vi "GetSpicyPizza.vi"(8 "error in (no error)":errorcluster, 11 "Waiter(Director) in":refnum<class "Waiter(Director).lvclass">) -> (0 "error out":errorcluster, 2 "Pizza":refnum<class "Pizza(Product).lvclass">, 3 "Waiter(Director) out":refnum<class "Waiter(Director).lvclass">)   [LabVIEW 2014, in "Waiter(Director).lvclass"]
uses:
  Waiter(Director).lvclass
  Pizza(Product)/Pizza(Product).lvclass
  ConcreteBuilder/SpicyPizzaBuilder/SpicyPizzaBuilder.lvclass
  Cook(builder)/PizzaBuilder(Builder).lvclass
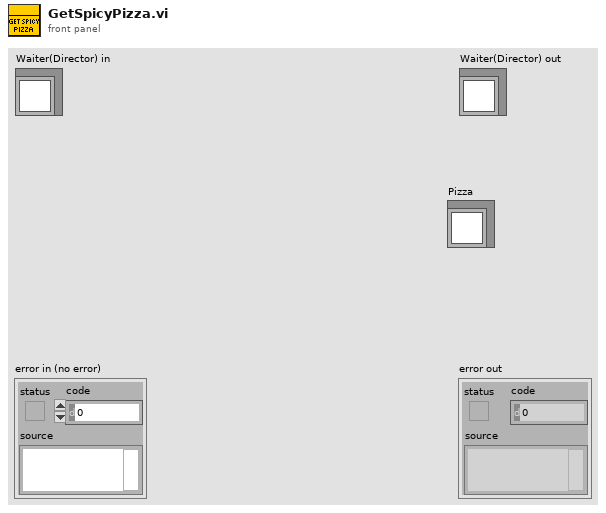
[diagram p1: front panel]
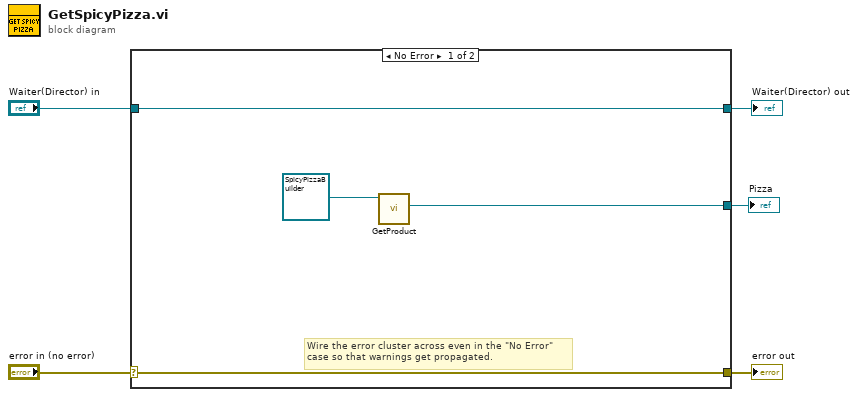
[diagram p0: block diagram]
diagram:
  n1 = case shown="No Error" "error in (no error)" {
    selector: "error in (no error)" -> [w8 w11]
    tunnel: [w8 w11] -> w4
    tunnel: [w9 w10] -> w2
    tunnel: "Waiter(Director) in" -> [w9 w10]
    tunnel: [w6 _] -> w1
    frame No Error {
      # "Wire the error cluster across even in the \"No Error\"\ncase so that warnings get propagated."
      n2 = call "GetProduct.vi"("PizzaBuilder(Builder) in"=refnum<class "SpicyPizzaBuilder.lvclass"> refnum ("SpicyPizzaBuilder")) -> ("Pizza"=w6:refnum<class "Pizza(Product).lvclass">)  [unwired: 8 in, 2 out]
    }
    frame Error {
    }
  }
  "error out" <- w4
  "Waiter(Director) out" <- w2
  "Pizza" <- w1
